vi "Pulse.vi"(10 "Input":bool, 11 "Rising Edge?":bool=TRUE) -> (2 "Output":bool)   [LabVIEW 2016]
panel:
  # "Sends out  a pulse only on the iteration the Input changes from false to true."
  # "Could be used when you want a joystick action to only happen once."
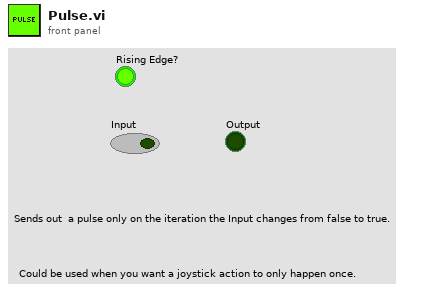
[diagram p1: front panel]
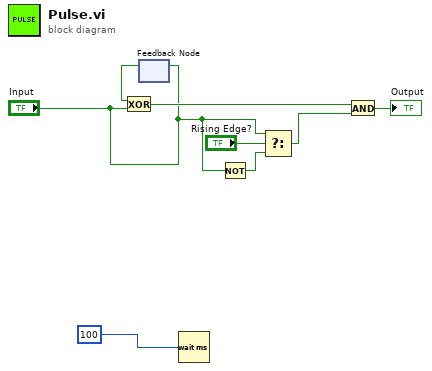
[diagram p0: block diagram]
diagram:
  n1 = feedback-in #1("Input") -> ()
  n2 = feedback #1() -> (w8:bool)  [unwired: 1 in]
  n3 = Exclusive Or(1:"Input", 2:w8) -> (0:w6:bool)
  n4 = Wait (ms)(milliseconds to wait=u32 100) -> ()  [unwired: 1 out]
  n5 = Not(x="Input") -> (.not. x?=w4:bool)
  n6 = Select(t="Input", s="Rising Edge?", f=w4) -> (s? t:f=w5:bool)
  n7 = And(x=w6, y=w5) -> (x .and. y?=→"Output":bool)
